vi "isAck.vi"(8 "error in (no error)":errorcluster, 10 "response":T1, 11 "BaseMessage in":refnum<class "BaseMessage.lvclass">) -> (0 "error out":errorcluster, 1 "isAck?":bool, 3 "BaseMessage out":refnum<class "BaseMessage.lvclass">)   [LabVIEW 2013, in "BaseMessage.lvclass"]
doc: "Returns TRUE if the response is an acknowledgement for the message. Overide in descendant message classes to add logic"
uses:
  BaseMessage.lvclass
  response.ctl
  driver_status.ctl
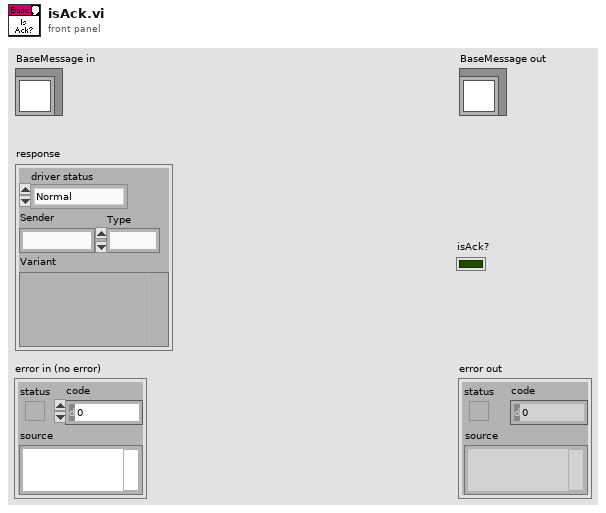
[diagram p1: front panel]
types:
  T1 = typedef "response.ctl" = cluster{"driver status":T2, "Sender":string, "Type":i32, "Variant":variant}
  T2 = typedef "driver_status.ctl" = enum16{"Normal", "Startup", "Connection lost", "Reconnected", "Timeout", "Idle", "Busy"}
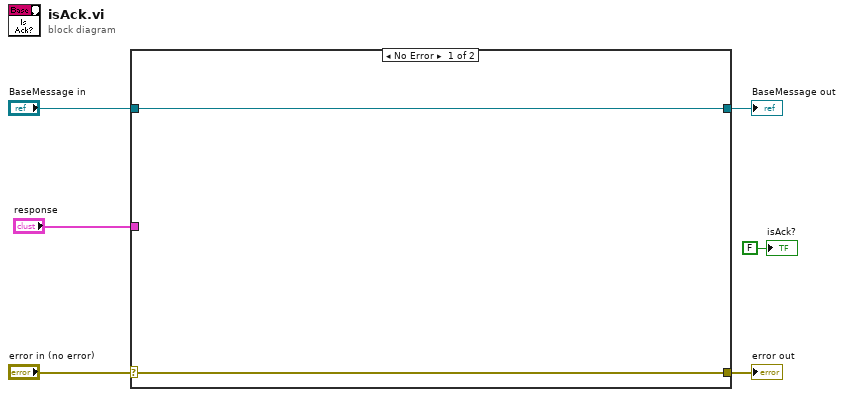
[diagram p0: block diagram]
diagram:
  n1 = case shown="No Error" "error in (no error)" {
    selector: "error in (no error)" -> [w7 w10]
    tunnel: [w7 w10] -> w5
    tunnel: [w8 w9] -> w3
    tunnel: "BaseMessage in" -> [w8 w9]
    tunnel: "response" -> [_ _]
    frame No Error {
    }
    frame Error {
    }
  }
  "error out" <- w5
  "BaseMessage out" <- w3
  "isAck?" <- FALSE ("found?")
